vi "test.vi"(0 "reference in":refnum<class "active object queue.lvclass">, 2 "MessageToProcess":string, 5 "error in (no error)":errorcluster) -> (14 "reference out":refnum<class "active object queue.lvclass">, 19 "error out":errorcluster)   [LabVIEW 2019, in "active object queue.lvclass"]
uses:
  active object queue.lvclass
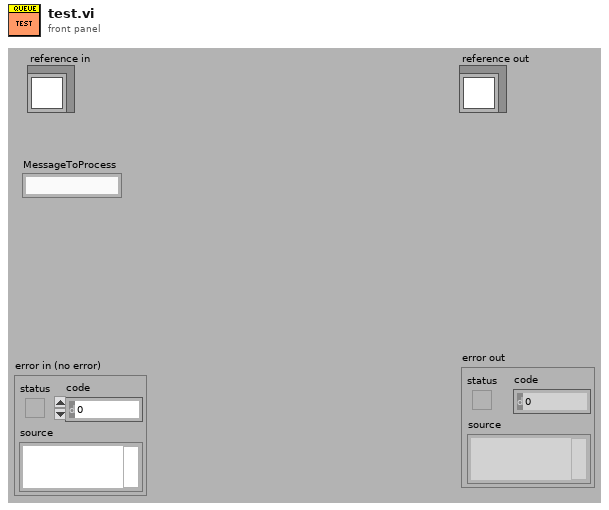
[diagram p1: front panel]
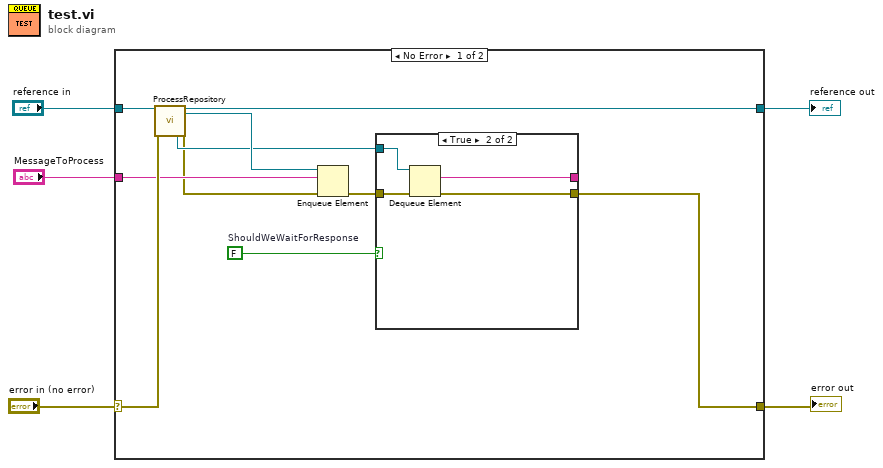
[diagram p0: block diagram]
diagram:
  n1 = case shown="No Error" "error in (no error)" {
    selector: "error in (no error)" -> [w15 w22]
    tunnel: [w6 w22] -> w4
    tunnel: [w13 w21] -> w2
    tunnel: "reference in" -> [w14 w21]
    tunnel: "MessageToProcess" -> [w11 _]
    frame No Error {
      w10 = FALSE  # ShouldWeWaitForResponse
      n2 = call "ProcessRepository.vi"("reference in"=w14, "error in (no error)"=w15) -> ("FromProcessQueue"=w8:refnum<queue>, "reference out"=w13:refnum<class "active object queue.lvclass">, "ToProcessQueue"=w12:refnum<queue>, "error out"=w7:errorcluster)  [unwired: 11 in, 3 out]
      n3 = Enqueue Element(queue=w12, element=w11, error in (no error)=w7) -> (error out=w9:errorcluster)  [unwired: 1 in, 2 out]
      n4 = case shown="True" w10 {
        tunnel: w9 -> [w16 w20]
        tunnel: w8 -> [_ w19]
        tunnel: [_ w18] -> _
        tunnel: [w16 w17] -> w6
        frame False {
        }
        frame True {
          n5 = Dequeue Element(queue=w19, error in (no error)=w20) -> (element=w18:string, error out=w17:errorcluster)  [unwired: 1 in, 2 out]
        }
      }
    }
    frame Error {
    }
  }
  "error out" <- w4
  "reference out" <- w2
